vi "Set V2 (SubVI).vi"(11 "Voltage Y":string) -> (3 "String":string)   [LabVIEW 2018]
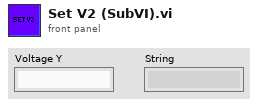
[diagram p1: front panel]
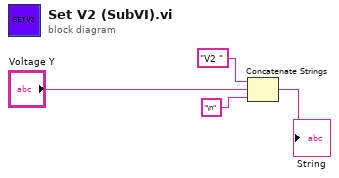
[diagram p0: block diagram]
diagram:
  n1 = Concatenate Strings("V2 ", "Voltage Y", "\n") -> (→"String":string)
